vi "Image File to 2D Image.vi"(8 "error in":errorcluster, 11 "Path":path) -> (0 "error out":errorcluster, 2 "image data":T1, 3 "2D Picture":picture)   [LabVIEW 2024, in "EQMF.lvlib" / "Graphic Utils.lvlib"]
uses:
  Graphic Utils.lvlib
  <vilib>/picture/picture.llb/imagedata.ctl
  Files/File Utils.lvlib
panel:
  # "Getr Image"
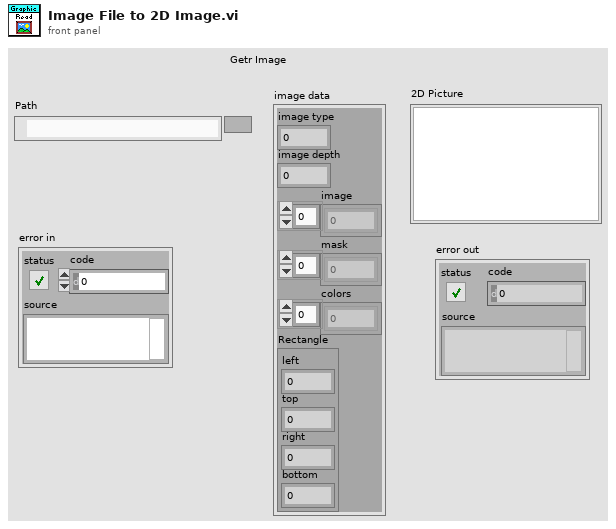
[diagram p1: front panel]
types:
  T1 = typedef "imagedata.ctl" = cluster{"image type":i32, "image depth":i32, "image":u8[], "mask":u8[], "colors":u32[], "Rectangle":cluster{"left":i16, "top":i16, "right":i16, "bottom":i16}}
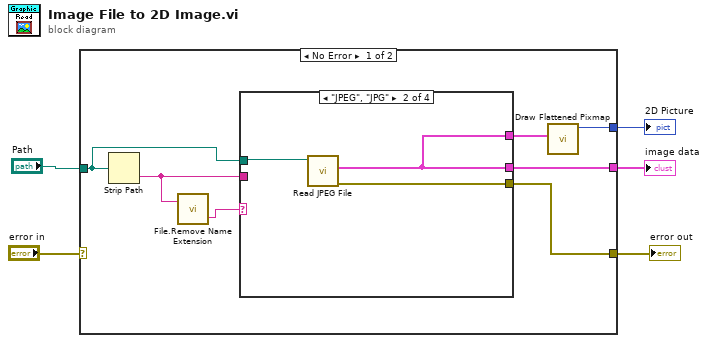
[diagram p0: block diagram]
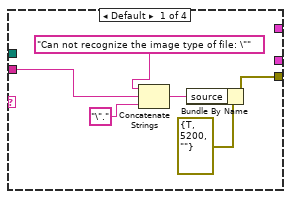
[diagram p2: hidden frame]
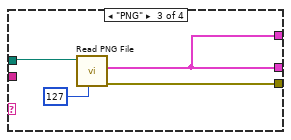
[diagram p3: hidden frame]
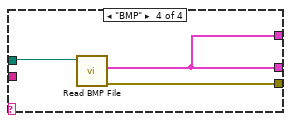
[diagram p4: hidden frame]
diagram:
  n1 = case shown="No Error" "error in" {
    selector: "error in" -> [_ w29]
    tunnel: "Path" -> [w9 _]
    tunnel: [w12 _] -> w4
    tunnel: [w10 w29] -> w3
    tunnel: [w6 _] -> w1
    frame No Error {
      n2 = Strip Path(path=w9) -> (name=w8:string)  [unwired: 1 out]
      n3 = call "File.Remove Name Extension.vi"("File Name"=w8) -> ("Ext"=w7:string)  [unwired: 1 in, 1 out]
      n4 = case shown="\"JPEG\", \"JPG\"" w7 {
        tunnel: w9 -> [_ w21 w25 w28]
        tunnel: [_ w19 w22 w26] -> w11
        tunnel: [w18 w20 w24 w27] -> w10
        tunnel: w8 -> [w15 _ _ _]
        tunnel: [_ w19 w22 w26] -> w6
        frame Default {
          n5 = Concatenate Strings("Can not recognize the image type of file: \"", w15, "\".") -> (w13:string)
          n6 = Bundle By Name(cluster=errorcluster {"status"=TRUE, "code"=5200, "source"=""} ("error constant"), "source"=w13) -> (w18:errorcluster)
        }
        frame "JPEG", "JPG" {
          n7 = call <vilib>:"Read JPEG File.vi"("path to JPEG file"=w21) -> ("error out"=w20:errorcluster, "image data"=w19:T1)  [unwired: 8 in, 1 out]
        }
        frame "PNG" {
          n8 = call <vilib>:"Read PNG File.vi"("Transparency Thresh"=u8 127, "path to PNG file"=w25) -> ("error out"=w24:errorcluster, "image data"=w22:T1)  [unwired: 7 in, 1 out]
        }
        frame "BMP" {
          n9 = call <vilib>:"Read BMP File.vi"("path to BMP file"=w28) -> ("error out"=w27:errorcluster, "image data"=w26:T1)  [unwired: 8 in, 1 out]
        }
      }
      n10 = call <vilib>:"Draw Flattened Pixmap.vi"("image data"=w11) -> ("new picture"=w12:picture)  [unwired: 8 in]
    }
    frame Error {
    }
  }
  "2D Picture" <- w4
  "error out" <- w3
  "image data" <- w1
